vi "Add Quotes for Array Input Database.vi"(11 "Array Input":string[](array[string])) -> (3 "Array Out":string[](array[string]))   [LabVIEW 2020]
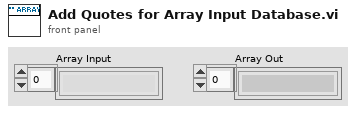
[diagram p1: front panel]
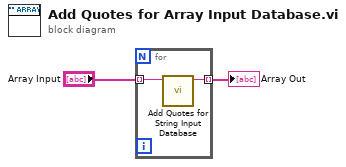
[diagram p0: block diagram]
diagram:
  n1 = for {
    tunnel: "Array Input" -> [w4] mode=indexing
    tunnel: [w3] -> w2 mode=indexing
    n2 = call "Add Quotes for String Input Database.vi"("String in"=w4) -> ("String Out"=w3:string)  [unwired: 10 in]
  }
  "Array Out" <- w2
